vi "判定范围并强制转换.vi"() -> ()   [LabVIEW 2018]
panel:
  out "字符串":string
  in  "停止":bool
  out "是否转换过？":bool
  out "转换结果":dbl
  in  "数值":dbl
  in  "下限":dbl
  in  "上限":dbl
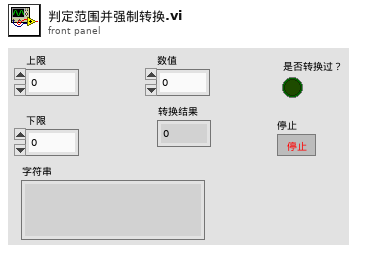
[diagram p1: front panel]
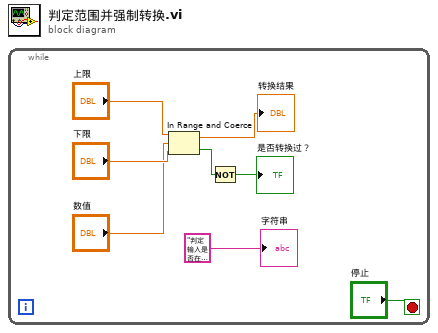
[diagram p0: block diagram]
diagram:
  n1 = while {
    stop <- "停止" stop-if-true
    n2 = In Range and Coerce(upper limit="上限", x="数值", lower limit="下限") -> (coerced(x)=→"转换结果":dbl, In Range?=w3:bool)
    n3 = Not(x=w3) -> (.not. x?=→"是否转换过？":bool)
    "字符串" <- "判定输入是否在范围内？\n是，输出输入值\n否，输出接近的上限或下限"
  }
